vi "2D_scanner.vi"(0 "pos-start_x":dbl=6.0, 5 "pos-start_y":dbl=6.0, 7 "image_size_x_um":dbl=6.0, 9 "frame_size_x_px":i32=50, 11 "pixel_dwell_ms":dbl=0.1 caption="Dwell time:", 12 "pos_start":enum32{"bottom-left", "center"}(ring), 13 "scan_direction":enum32{"0", "1"}(radio)=enum."1" caption="Scan direction:") -> (6 "image_out":dbl[][](array[numeric]))   [LabVIEW 2018]
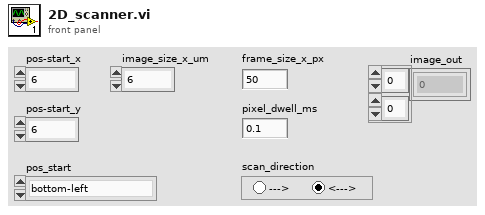
[diagram p1: front panel]
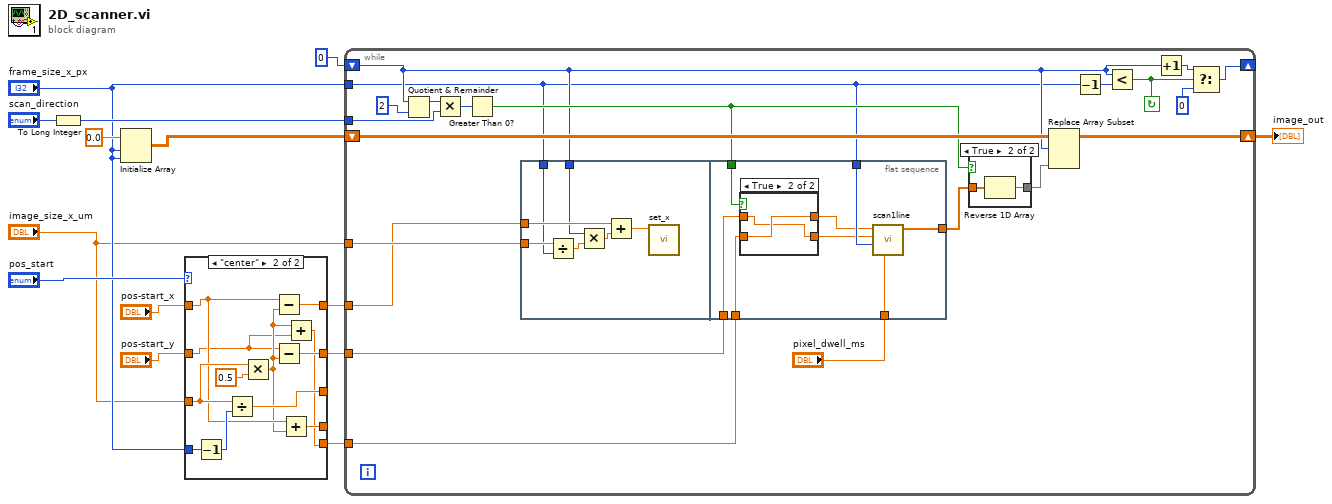
[diagram p0: block diagram]
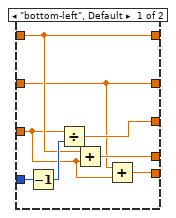
[diagram p2: hidden frame]
diagram:
  n1 = To Long Integer(number="scan_direction") -> (32bit integer=w10:i32)
  n2 = Initialize Array(0.0 ("element"), "frame_size_x_px", "frame_size_x_px") -> (w12:dbl[][])
  n3 = case shown="\"center\"" "pos_start" {
    tunnel: "pos-start_x" -> [w19 w28]
    tunnel: "pos-start_y" -> [w16 w25]
    tunnel: "image_size_x_um" -> [w17 w32]
    tunnel: [w19 w29] -> w2
    tunnel: [w16 w30] -> w1
    tunnel: [w21 w33] -> _
    tunnel: [w20 w27] -> _
    tunnel: [w18 w24] -> w5
    tunnel: "frame_size_x_px" -> [w15 w23]
    frame "bottom-left", Default {
      n4 = Decrement(x=w15) -> (x-1=w22:i32)
      n5 = Divide(x=w17, y=w22) -> (x/y=w21:dbl)
      n6 = Add(x=w19, y=w17) -> (x+y=w20:dbl)
      n7 = Add(x=w16, y=w17) -> (x+y=w18:dbl)
    }
    frame "center" {
      n8 = Decrement(x=w23) -> (x-1=w34:i32)
      n9 = Divide(x=w32, y=w34) -> (x/y=w33:dbl)
      n10 = Multiply(x=w32, y=0.5) -> (x*y=w26:dbl)
      n11 = Subtract(x=w28, y=w26) -> (x-y=w29:dbl)
      n12 = Subtract(x=w25, y=w26) -> (x-y=w30:dbl)
      n13 = Add(x=w28, y=w26) -> (x+y=w27:dbl)
      n14 = Add(x=w26, y=w25) -> (x+y=w24:dbl)
    }
  }
  n15 = while {
    shift-right: [w38] -> w9
    shift-left: w12 -> [w55]
    shift-right: [w54] -> _
    shift-left: 0 -> [w43]
    tunnel: "frame_size_x_px" -> [w42]
    tunnel: w10 -> [w44]
    tunnel: "image_size_x_um" -> [w41]
    tunnel: w5 -> [w37]
    tunnel: w2 -> [w36]
    tunnel: w1 -> [w35]
    stop <- w39 continue-if-true
    n16 = Quotient & Remainder(x=w43, y=2) -> (x-y*floor(x/y)=w49:i32)  [unwired: 1 out]
    n17 = Multiply(x=w49, y=w44) -> (x*y=w48:i32)
    n18 = Greater Than 0?(x=w48) -> (x > 0?=w45:bool)
    n19 = flat-sequence {
      tunnel: w36 -> [w62]
      tunnel: w43 -> [w60]
      tunnel: w41 -> [w58]
      tunnel: w42 -> [w57]
      tunnel: [w70] -> w47
      tunnel: w42 -> [w69]
      tunnel: w45 -> [w66]
      tunnel: w35 -> [w65]
      tunnel: w37 -> [w64]
      tunnel: "pixel_dwell_ms" -> [w63]
      frame #0 {
        n20 = Divide(x=w58, y=w57) -> (x/y=w59:dbl)
        n21 = Multiply(x=w60, y=w59) -> (x*y=w61:dbl)
        n22 = Add(x=w62, y=w61) -> (x+y=w56:dbl)
        n23 = call "set_x.vi"("x_value_um"=w56) -> ()  [unwired: 10 in, 1 out]
      }
      frame #1 {
        n24 = case shown="True" w66 {
          tunnel: [w71 w74] -> w68
          tunnel: [w72 w73] -> w67
          tunnel: w64 -> [w72 w74]
          tunnel: w65 -> [w71 w73]
          frame False {
          }
          frame True {
          }
        }
        n25 = call "scan1line.vi"("dwell_time_ms"=w63, "q_pixels"=w69, "y_end"=w67, "y_start"=w68) -> ("histogram plot"=w70:dbl[])  [unwired: 6 in, 1 out]
      }
    }
    n26 = case shown="True" w45 {
      tunnel: w47 -> [w75 w77]
      tunnel: [w75 w76] -> w46
      frame False {
      }
      frame True {
        n27 = Reverse 1D Array(array=w77) -> (reversed array=w76:dbl[])
      }
    }
    n28 = Replace Array Subset(array=w55, new element=w46, index (row)=w43) -> (w38:dbl[][])  [unwired: 1 in]
    n29 = Decrement(x=w42) -> (x-1=w51:i32)
    n30 = Less?(x=w43, y=w51) -> (x < y?=w39:bool)
    n31 = Increment(x=w43) -> (x+1=w53:i32)
    n32 = Select(t=w53, s=w39, f=0) -> (s? t:f=w54:i32)
  }
  "image_out" <- w9
